vi "Detect Intake Object.vi"(11 "Refnum in":T1(plugin-control)) -> (3 "Refnum out":T1(plugin-control))   [LabVIEW 2014]
uses:
  <vilib>/vision/NI_Vision_Development_Module.lvlib
panel:
  out "String":string
  in  "Sat Thresh":dbl
  in  "Luma Thresh":dbl
  out "Sat":dbl format="%.6f"
  out "Luma":dbl format="%.6f"
  out "Boolean 2":bool
  out "B":dbl
  out "G":dbl
  out "Boolean":bool
  out "R":dbl
  out "Red or Hue Plane out":T1(plugin-control)
  in  "Exam Zone Offset Y":dbl
  in  "Exam Zone Offset X":dbl
  out "Image Dst Out":T1(plugin-control)
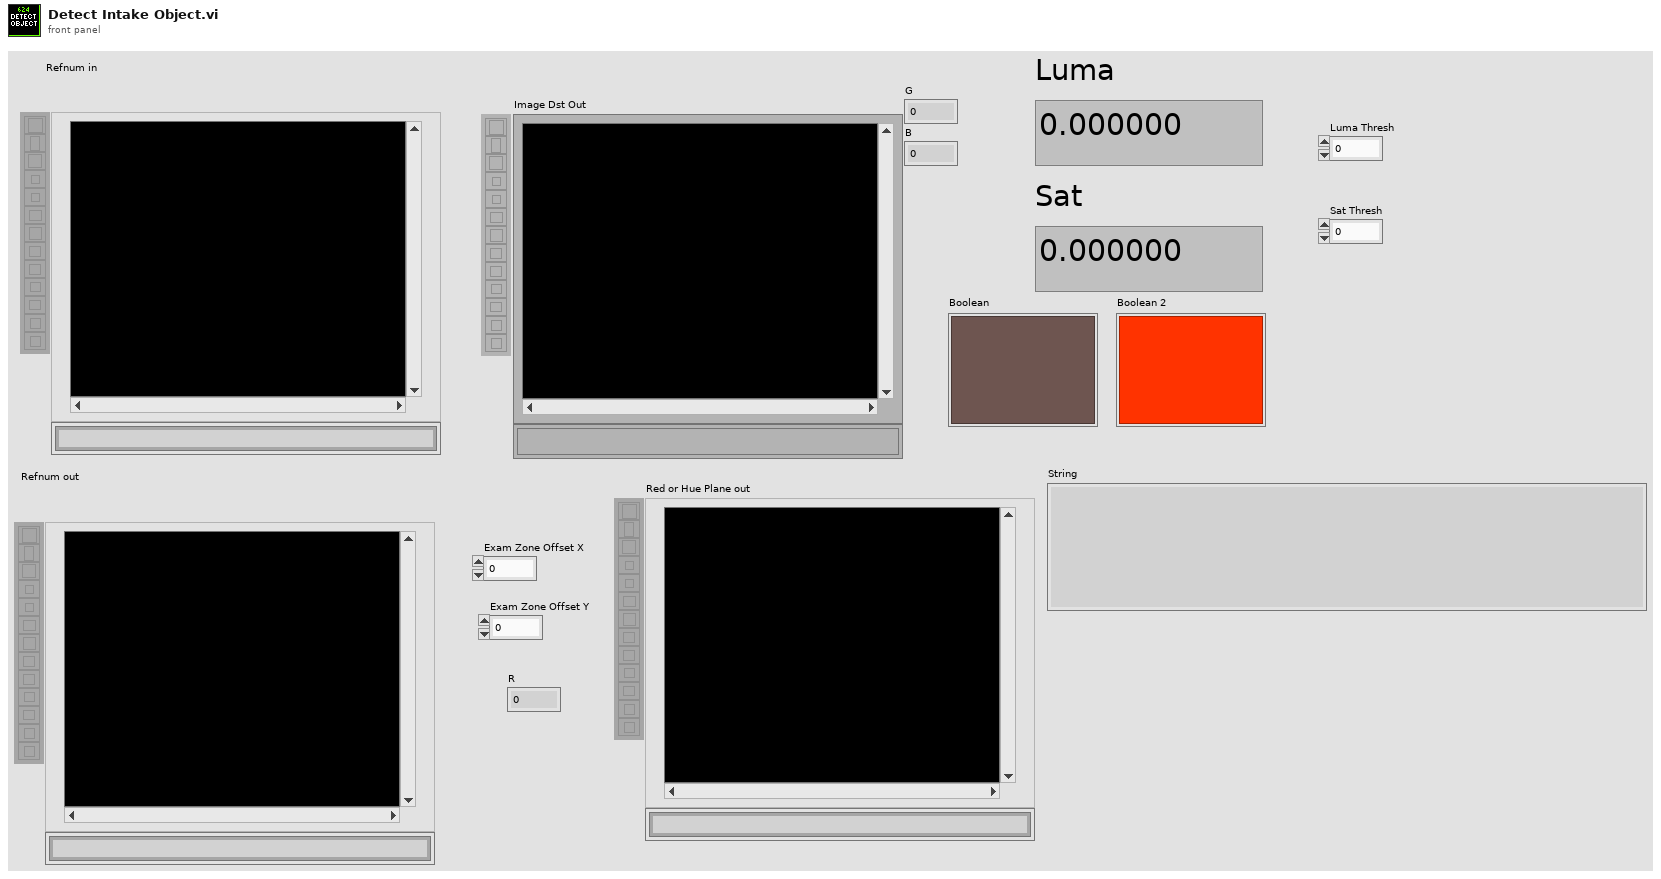
[diagram p1: front panel]
types:
  T1 = typedef "IMAQ Image.ctl" = refnum<image>
  T2 = typedef "Image Type" = u32
  T3 = cluster{"[0]":i32, "[1]":i32, "[2]":i32, "[3]":i32}
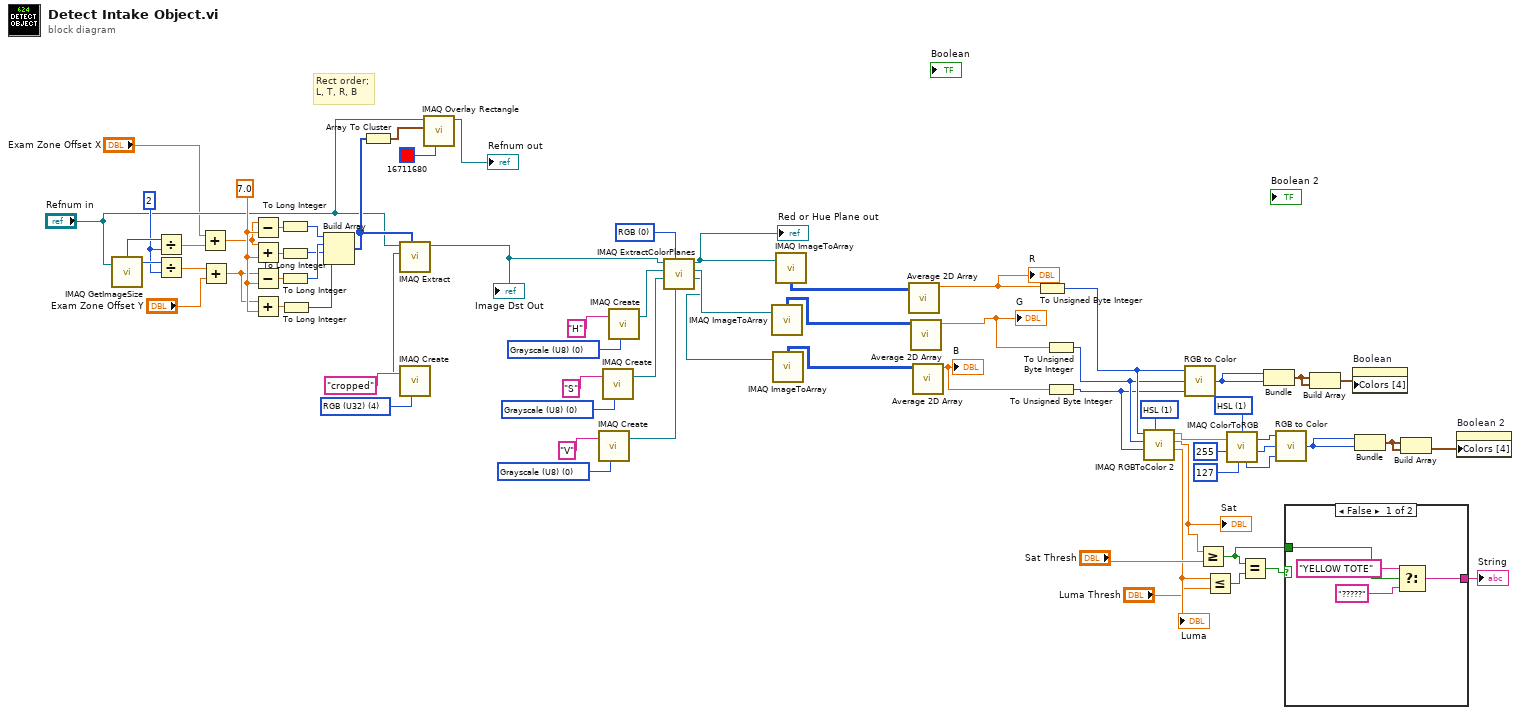
[diagram p0: block diagram]
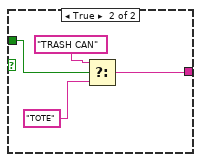
[diagram p2: hidden frame]
diagram:
  w17 = u16 1 items=["RGB", "HSL", "HSV", "HSI"] ("Color Mode")
  w18 = u16 1 items=["RGB", "HSL", "HSV", "HSI", "CIE L*a*b*", "CIE XYZ"] ("Color Mode")
  w37 = T2 0 items=["Grayscale (U8)", "Grayscale (I16)", "Grayscale (SGL)", "Complex (CSG)", "RGB (U32)", "HSL (U32)", "RGB (U64)", "Grayscale (U16)"] ("Image Type")
  w39 = T2 0 items=["Grayscale (U8)", "Grayscale (I16)", "Grayscale (SGL)", "Complex (CSG)", "RGB (U32)", "HSL (U32)", "RGB (U64)", "Grayscale (U16)"] ("Image Type")
  w43 = T2 0 items=["Grayscale (U8)", "Grayscale (I16)", "Grayscale (SGL)", "Complex (CSG)", "RGB (U32)", "HSL (U32)", "RGB (U64)", "Grayscale (U16)"] ("Image Type")
  w44 = u16 0 items=["RGB", "HSL", "HSV", "HSI"] ("Color Mode")
  w59 = T2 4 items=["Grayscale (U8)", "Grayscale (I16)", "Grayscale (SGL)", "Complex (CSG)", "RGB (U32)", "HSL (U32)", "RGB (U64)", "Grayscale (U16)"] ("Image Type")
  w68 = 7.0
  w69 = 2 ("y")
  # "Rect order;\nL, T, R, B"
  n1 = call "IMAQ GetImageSize"("Image"="Refnum in") -> ("Y Resolution"=w70:i32, "X Resolution"=w71:i32)  [unwired: 3 in, 1 out]
  n2 = Divide(x=w71, y=w69) -> (x/y=w51:dbl)
  n3 = Divide(x=w70, y=w69) -> (x/y=w49:dbl)
  n4 = Add(x="Exam Zone Offset X", y=w51) -> (x+y=w46:dbl)
  n5 = Add(x=w49, y="Exam Zone Offset Y") -> (x+y=w47:dbl)
  n6 = Subtract(x=w46, y=w68) -> (x-y=w67:dbl)
  n7 = Add(x=w46, y=w68) -> (x+y=w57:dbl)
  n8 = Subtract(x=w47, y=w68) -> (x-y=w66:dbl)
  n9 = Add(x=w47, y=w68) -> (x+y=w65:dbl)
  n10 = To Long Integer(number=w67) -> (32bit integer=w64:i32)
  n11 = To Long Integer(number=w57) -> (32bit integer=w62:i32)
  n12 = To Long Integer(number=w66) -> (32bit integer=w63:i32)
  n13 = To Long Integer(number=w65) -> (32bit integer=w61:i32)
  n14 = Build Array(w64, w63, w62, w61) -> (w56:i32[])
  n15 = Array To Cluster(array=w56) -> (cluster=w55:T3)
  n16 = call "IMAQ Create"("Image Name"="cropped", "Image Type"=w59) -> ("New Image"=w58:T1)  [unwired: 3 in, 1 out]
  n17 = call "IMAQ Extract"("Optional Rectangle"=w56, "Image Dst"=w58, "Image Src"="Refnum in") -> ("Image Dst Out"=w45:T1)  [unwired: 7 in, 1 out]
  "Image Dst Out" <- w45
  n18 = call "IMAQ Overlay Rectangle"("Color"=u32 16711680, "Rectangle"=w55, "Image"="Refnum in") -> ("Image Out"=→"Refnum out":T1)  [unwired: 7 in, 1 out]
  n19 = call "IMAQ Create"("Image Name"="V", "Image Type"=w37) -> ("New Image"=w35:T1)  [unwired: 3 in, 1 out]
  n20 = call "IMAQ Create"("Image Name"="S", "Image Type"=w39) -> ("New Image"=w38:T1)  [unwired: 3 in, 1 out]
  n21 = call "IMAQ Create"("Image Name"="H", "Image Type"=w43) -> ("New Image"=w41:T1)  [unwired: 3 in, 1 out]
  n22 = call "IMAQ ExtractColorPlanes"("Blue or Luma or Val or Inten Plane"=w35, "Color Mode"=w44, "Green or Sat Plane"=w38, "Red or Hue Plane"=w41, "Image Src"=w45) -> ("Blue or Luma or Val or Inten Plane out"=w28:T1, "Green or Sat Plane out"=w29:T1, "Red or Hue Plane out"=w34:T1)  [unwired: 3 in, 1 out]
  "Red or Hue Plane out" <- w34
  n23 = call "IMAQ ImageToArray"("Image"=w29) -> ("Image Pixels (U8)"=w27:u8[][])  [unwired: 3 in, 4 out]
  n24 = call "IMAQ ImageToArray"("Image"=w28) -> ("Image Pixels (U8)"=w26:u8[][])  [unwired: 3 in, 4 out]
  n25 = call "IMAQ ImageToArray"("Image"=w34) -> ("Image Pixels (U8)"=w33:u8[][])  [unwired: 3 in, 4 out]
  n26 = call "Average 2D Array.vi"("Image Pixels (U8)"=w33) -> ("Numeric"=w32:dbl)  [unwired: 10 in]
  "R" <- w32
  n27 = call "Average 2D Array.vi"("Image Pixels (U8)"=w27) -> ("Numeric"=w25:dbl)  [unwired: 10 in]
  "G" <- w25
  n28 = call "Average 2D Array.vi"("Image Pixels (U8)"=w26) -> ("Numeric"=w24:dbl)  [unwired: 10 in]
  "B" <- w24
  n29 = To Unsigned Byte Integer(number=w32) -> (unsigned 8bit integer=w22:u8)
  n30 = To Unsigned Byte Integer(number=w25) -> (unsigned 8bit integer=w21:u8)
  n31 = To Unsigned Byte Integer(number=w24) -> (unsigned 8bit integer=w20:u8)
  n32 = call "IMAQ RGBToColor 2"("Color Mode"=w18, "Blue value"=w20, "Green value"=w21, "Red value"=w22) -> ("Blue or Luma or Val or Inten or Z or b*value"=w7:dbl, "Green or Sat or Y or a* value"=w8:dbl, "Red or Hue or X or L* value"=w19:dbl)  [unwired: 4 in, 1 out]
  "Luma" <- w7
  "Sat" <- w8
  n33 = call <vilib>:"RGB to Color.vi"("B"=w20, "G"=w21, "R"=w22) -> ("Color"=w23:u32)
  n34 = Greater Or Equal?(x=w8, y="Sat Thresh") -> (x >= y?=w2:bool)
  n35 = Less Or Equal?(x=w7, y="Luma Thresh") -> (x <= y?=w4:bool)
  n36 = call "IMAQ ColorToRGB"("Green or Sat value"=u8 255, "Blue or Luma or Val or Inten value"=u8 127, "Red or Hue value"=w19, "Color Mode"=w17) -> ("Blue value"=w10:u8, "Green value"=w11:u8, "Red value"=w12:u8)  [unwired: 1 in, 1 out]
  n37 = Equal?(x=w2, y=w4) -> (x = y?=w3:bool)
  n38 = Bundle("Color"=w23, "Color"=w23) -> (w31:cluster{"Color":u32, "Color":u32})  [unwired: 1 in]
  n39 = call <vilib>:"RGB to Color.vi"("B"=w10, "G"=w11, "R"=w12) -> ("Color"=w14:u32)
  n40 = case shown="False" w3 {
    tunnel: w2 -> [w75 w76]
    tunnel: [w74 w77] -> w1
    frame False {
      n41 = Select(t="YELLOW TOTE", s=w75, f="?????") -> (s? t:f=w74:string)
    }
    frame True {
      n42 = Select(t="TRASH CAN", s=w76, f="TOTE") -> (s? t:f=w77:string)
    }
  }
  "String" <- w1
  n43 = Build Array(w31, w31) -> (w30:cluster{"Color":u32, "Color":u32}[])
  n44 = property on="Boolean" class="Bool (strict)"("Colors [4]"=w30) -> ()  [unwired: 2 in, 2 out]
  n45 = Bundle("Color"=w14, "Color"=w14) -> (w13:cluster{"Color":u32, "Color":u32})  [unwired: 1 in]
  n46 = Build Array(w13, w13) -> (w5:cluster{"Color":u32, "Color":u32}[])
  n47 = property on="Boolean 2" class="Bool (strict)"("Colors [4]"=w5) -> ()  [unwired: 2 in, 2 out]
